vi "Clear Plugins.vi"(8 "error in (no error)":errorcluster, 11 "Execution UI in":refnum<class "Execution UI.lvclass">) -> (0 "error out":errorcluster, 3 "Execution UI out":refnum<class "Execution UI.lvclass">)   [LabVIEW 2020, in "Execution UI.lvclass"]
uses:
  Execution UI.lvclass
  Execution UI.lvclass/Execution UI.ctl
  Framework/Plugin/Plugin.lvclass
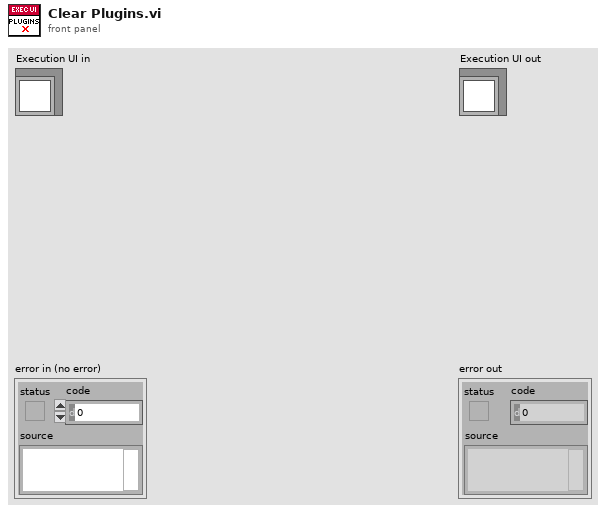
[diagram p1: front panel]
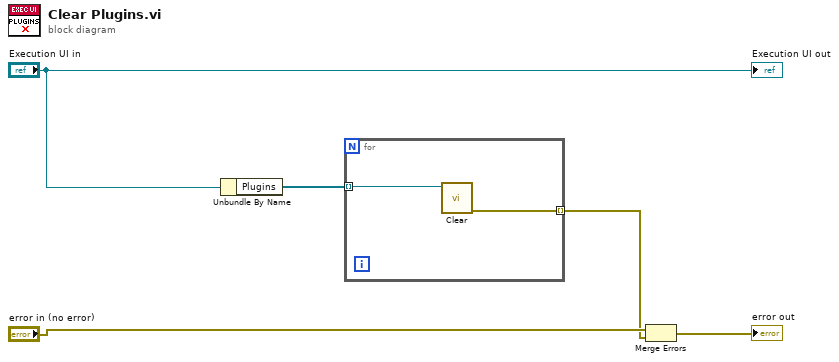
[diagram p0: block diagram]
diagram:
  n1 = Unbundle By Name("Execution UI in") -> ("Plugins"=w4:refnum<class "Plugin.lvclass">[])
  n2 = for {
    tunnel: w4 -> [w6] mode=indexing
    tunnel: [w7] -> w2 mode=indexing
    n3 = call-dynamic "Clear.vi"("Plugin in"=w6) -> ("error out"=w7:errorcluster)  [unwired: 10 in]
  }
  n4 = Merge Errors("error in (no error)", w2) -> (→"error out":errorcluster)
  "Execution UI out" <- "Execution UI in"
